vi "execute_comm.vi"(8 "error in (no error)":errorcluster, 10 "Command":string, 11 "VISA In":refnum<visa-resource-name>) -> (0 "error out":errorcluster, 2 "Return Value":string, 3 "VISA Out":refnum<visa-resource-name>)   [LabVIEW 2011]
uses:
  delay_time.vi
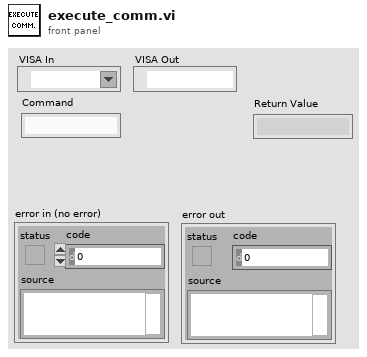
[diagram p1: front panel]
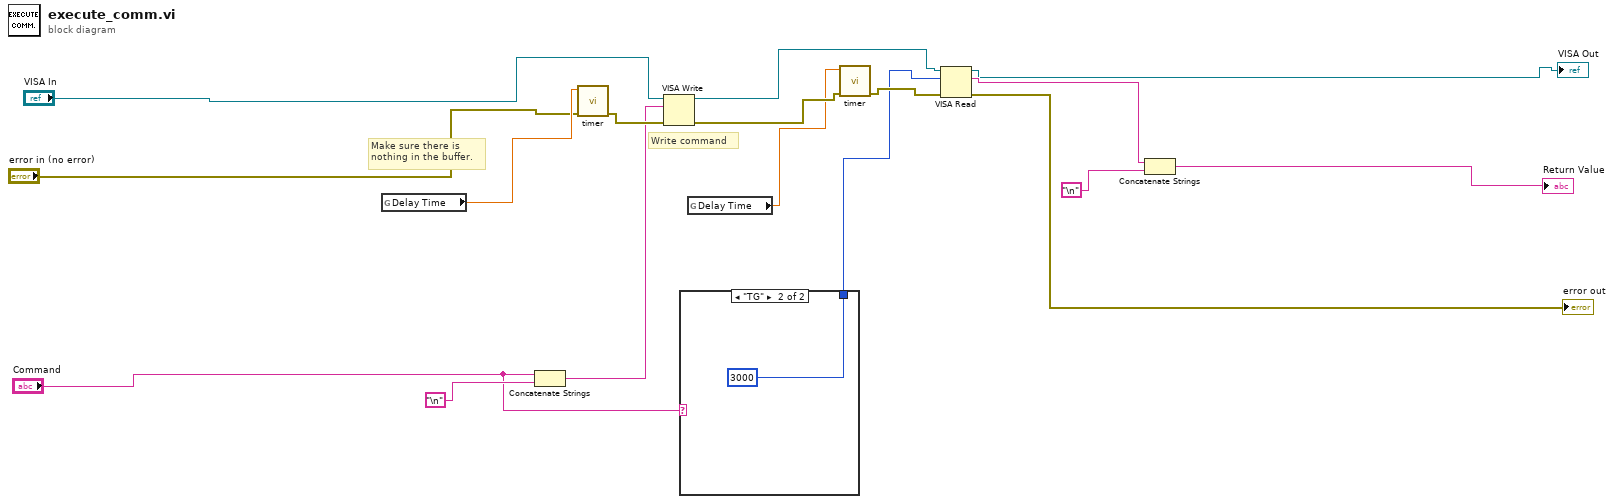
[diagram p0: block diagram]
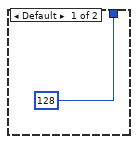
[diagram p2: hidden frame]
diagram:
  # "Write command"
  # "Make sure there is\nnothing in the buffer."
  n1 = global read "delay_time.vi" "Delay Time"() -> (w15:dbl)
  n2 = Concatenate Strings("Command", "\n") -> (w3:string)
  n3 = call "timer.vi"("error in (no error)"="error in (no error)", "Delay Time"=w15) -> ("error out"=w16:errorcluster)  [unwired: 9 in]
  n4 = VISA Write(VISA resource name="VISA In", write buffer=w3, error in (no error)=w16) -> (VISA resource name out=w11:refnum<visa-resource-name>, error out=w14:errorcluster)  [unwired: 1 out]
  n5 = case shown="\"TG\"" "Command" {
    tunnel: [128 3000] -> w2
    frame Default {
    }
    frame "TG" {
    }
  }
  n6 = global read "delay_time.vi" "Delay Time"() -> (w13:dbl)
  n7 = call "timer.vi"("error in (no error)"=w14, "Delay Time"=w13) -> ("error out"=w12:errorcluster)  [unwired: 9 in]
  n8 = VISA Read(VISA resource name=w11, byte count=w2, error in (no error)=w12) -> (VISA resource name out=→"VISA Out":refnum<visa-resource-name>, read buffer=w9:string, error out=→"error out":errorcluster)  [unwired: 1 out]
  n9 = Concatenate Strings(w9, "\n") -> (→"Return Value":string)
